vi "ITM10_alarm.vi"(3 "enabled":bool=TRUE, 5 "T_hihi":dbl=85.0 format="%.1f", 7 "T_hi":dbl=78.0 format="%.1f", 8 "time_last_alarm_in":timestamp, 10 "readout_status":bool=TRUE, 11 "value_array":dbl[](array[numeric])) -> (0 "time_last_alarm_out":timestamp, 2 "alarm_status":u32(colorbox))   [LabVIEW 2019]
panel:
  out "message":string
  in  "interval":dbl=3600.0
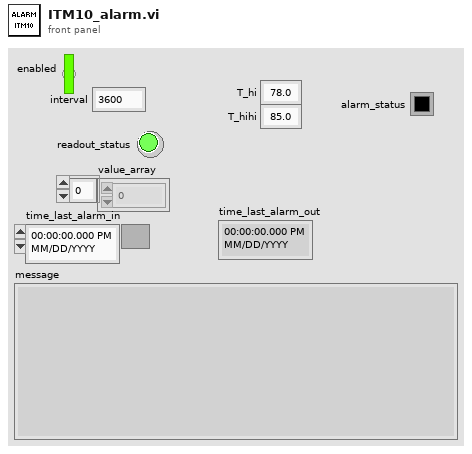
[diagram p1: front panel]
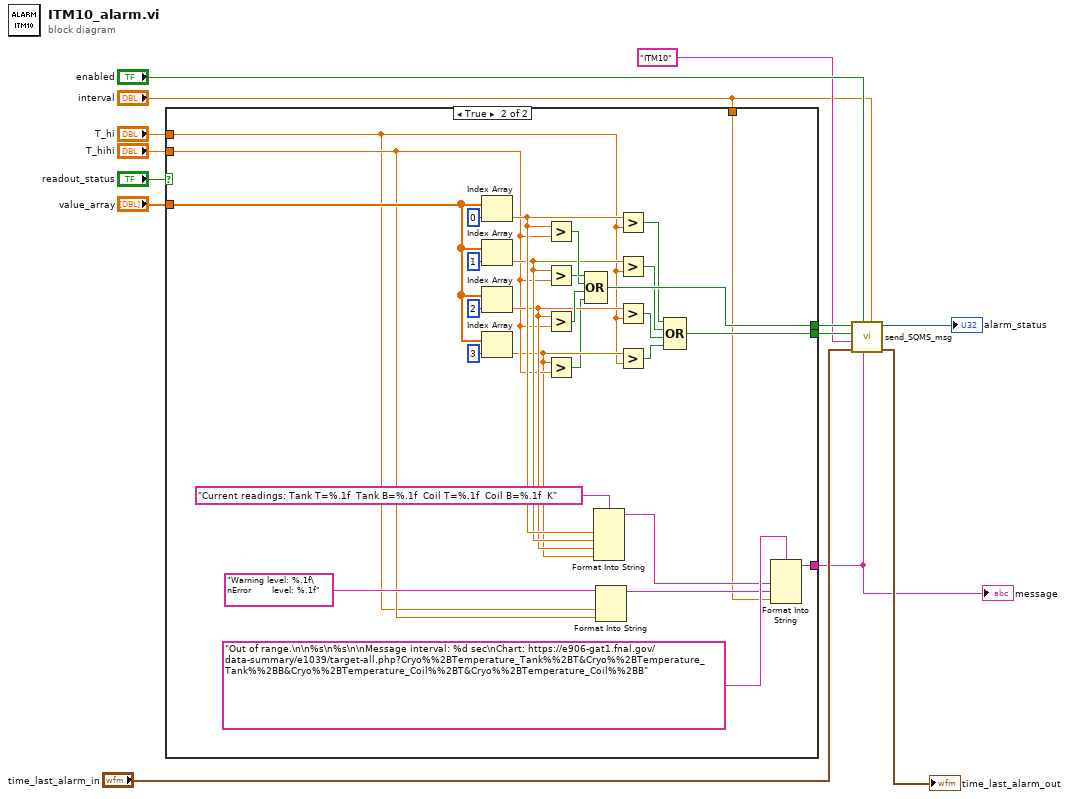
[diagram p0: block diagram]
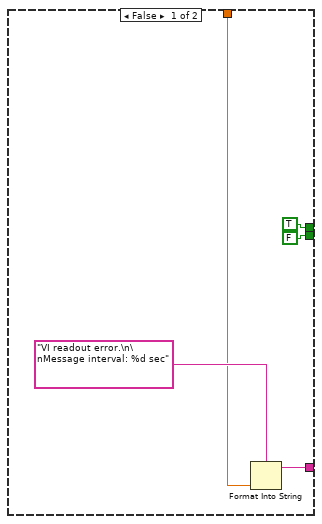
[diagram p2: hidden frame]
diagram:
  n1 = case shown="True" "readout_status" {
    tunnel: [TRUE w40] -> w12
    tunnel: [FALSE w36] -> w11
    tunnel: "value_array" -> [_ w34]
    tunnel: "T_hi" -> [_ w19]
    tunnel: "T_hihi" -> [_ w23]
    tunnel: "interval" -> [w14 w25]
    tunnel: [w15 w24] -> w3
    frame False {
      n2 = Format Into String(format string="VI readout error.\n\nMessage interval: %d sec" ("msg"), w14) -> (resulting string=w15:string)  [unwired: 2 in, 1 out]
    }
    frame True {
      n3 = Index Array(array=w34, index=0) -> (element=w32:dbl)
      n4 = Index Array(array=w34, index=1) -> (element=w31:dbl)
      n5 = Index Array(array=w34, index=2) -> (element=w30:dbl)
      n6 = Index Array(array=w34, index=3) -> (element=w22:dbl)
      n7 = Greater?(x=w32, y=w23) -> (0:w43:bool)
      n8 = Greater?(x=w31, y=w23) -> (0:w42:bool)
      n9 = Greater?(x=w30, y=w23) -> (0:w41:bool)
      n10 = Greater?(x=w22, y=w23) -> (0:w21:bool)
      n11 = Compound Arithmetic op=OR(w43, w42, w41, w21) -> (w40:bool)
      n12 = Format Into String(format string="Current readings: Tank T=%.1f  Tank B=%.1f  Coil T=%.1f  Coil B=%.1f  K" ("msg"), w32, w31, w30, w22) -> (resulting string=w27:string)  [unwired: 2 in, 1 out]
      n13 = Format Into String(format string="Warning level: %.1f\nError       level: %.1f" ("msg"), w19, w23) -> (resulting string=w26:string)  [unwired: 2 in, 1 out]
      n14 = Greater?(x=w32, y=w19) -> (0:w39:bool)
      n15 = Greater?(x=w31, y=w19) -> (0:w38:bool)
      n16 = Greater?(x=w30, y=w19) -> (0:w37:bool)
      n17 = Greater?(x=w22, y=w19) -> (0:w20:bool)
      n18 = Compound Arithmetic op=OR(w39, w38, w37, w20) -> (w36:bool)
      n19 = Format Into String(format string="Out of range.\n\n%s\n%s\n\nMessage interval: %d sec\nChart: https://e906-gat1.fnal.gov/data-summary/e1039/target-all.php?Cryo%%2BTemperature_Tank%%2BT&Cryo%%2BTemperature_Tank%%2BB&Cryo%%2BTemperature_Coil%%2BT&Cryo%%2BTemperature_Coil%%2BB" ("msg"), w27, w26, w25) -> (resulting string=w24:string)  [unwired: 2 in, 1 out]
    }
  }
  "message" <- w3
  n20 = call "send_SQMS_msg.vi"("alarm_interval"="interval", "msg"=w3, "enabled"="enabled", "time_last_alarm_in"="time_last_alarm_in", "title"="ITM10", "warning"=w11, "error"=w12) -> ("time_last_alarm_out"=→"time_last_alarm_out":timestamp, "alarm_status"=→"alarm_status":u32)  [unwired: 2 in, 1 out]
